vi "VI-File-Explorer.vi"() -> ()   [LabVIEW 2016, in "vi_lib.lvlib"]
uses:
  vi_lib.lvlib
  clLabview/clLabview.lvclass
  clFile/clFile.lvclass
panel:
  in  "new VI-Lib Password":string
  in  "Update LV-Lib Password":bool
  out "File is protected?":bool=TRUE
  out "LV-Lib password (Hex)":string
  out "Icon":picture
  out "busy (*)":bool
  out "Salt (Hex)":string
  out "MD5-Hash 2 (Hex)":string
  out "MD5-Hash 1 (Hex)":string
  out "saving done":bool
  in  "Save":bool
  in  "Open":bool
  in  "stop":bool
  out "flags":i32 step=1
  out "stage":u8(ring) items=["development", "alpha", "beta", "release"]
  out "build":u8 step=1
  out "bugfix":u8 step=1
  out "minor":u8 max=99 step=1
  out "major":u8=3 min=1 max=99 step=1
  out "version info":string
  out "version text":string
  in  "save to":path=path "D:/labview/file_in_(free).vi"
  in  "new File Password":string
  in  "open from":path
  out "MD5 password (Hex)":string
  # "File password [BDPW]"
  # "VI-File Explorer v.0.9"
  # "by Thomas Zeugner"
  # "Please report bugs and comments to: TomSoftware@gmx.de"
  # "Open"
  # "for LV-Version >= 8"
  # "for LV-Version >= 12"
  # "Save"
  # "File propertys [LVSR]"
  # "File version [vers]"
  # "(*) This is a \"brute force\" version to calc the password Salt, \n      so it might take up to 30sec."
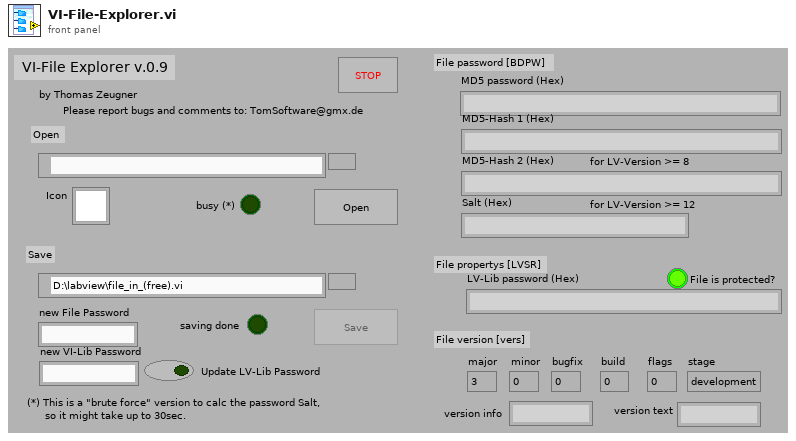
[diagram p1: front panel]
types:
  T1 = enum8{"Enabled", "Disabled", "Disabled and Grayed Out"}
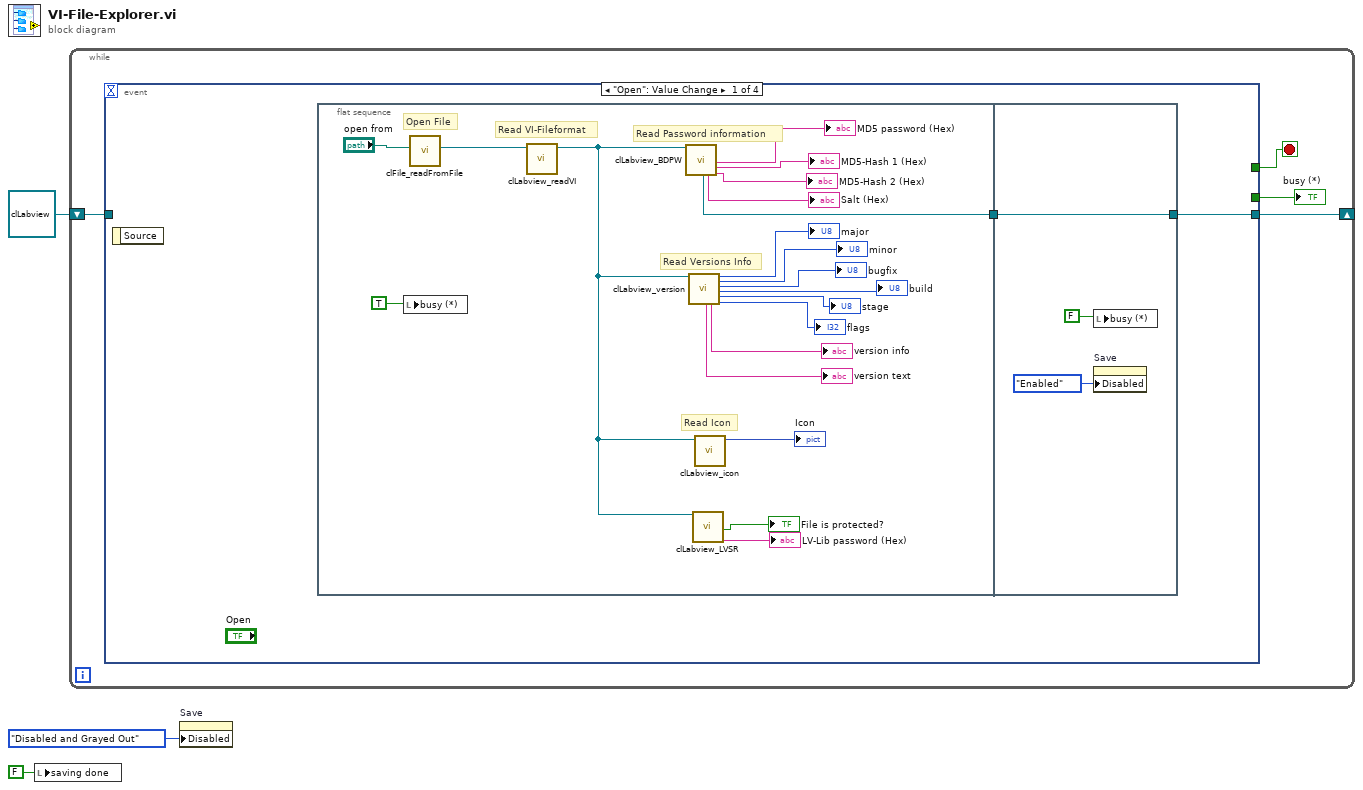
[diagram p0: block diagram]
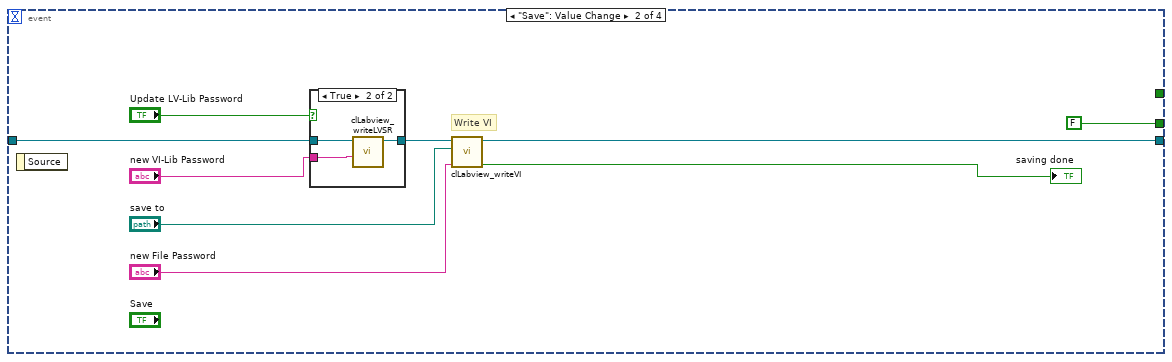
[diagram p2: hidden frame]
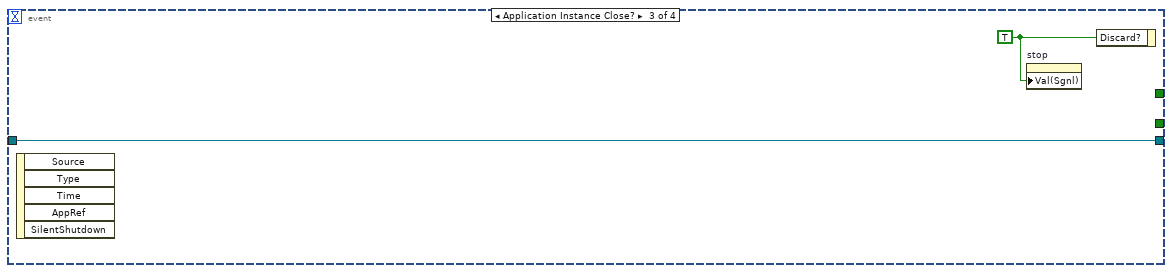
[diagram p4: hidden frame]
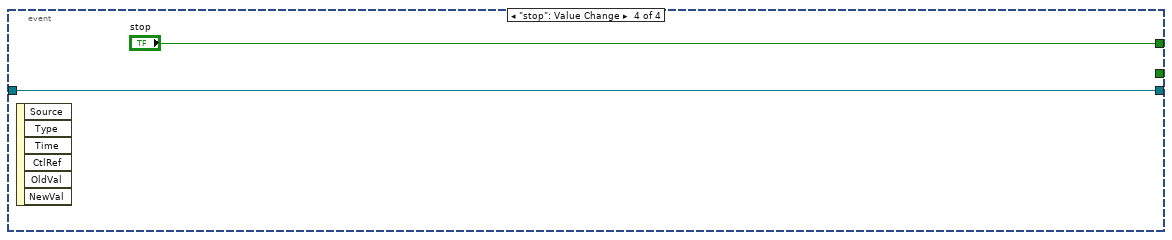
[diagram p5: hidden frame]
diagram:
  n1 = local write "saving done"(FALSE ("saving done")) -> ()
  n2 = while {
    shift-right: [w6] -> _
    shift-left: refnum<class "clLabview.lvclass"> refnum ("vi_lib.lvlib:clLabview.lvclass 2") -> [w7]
    stop <- w4 stop-if-true
    n3 = event shown="[0] \"Open\": Value Change" {
      selector: _ -> [_ _ _ _]
      dyn-events: _ -> [_ _ _ _]
      timeout: _ -> [_ _ _ _]
      tunnel: w7 -> [_ w35 w46 w48]
      tunnel: [w8 w34 w46 w48] -> w6
      tunnel: [_ FALSE ("busy") _ _] -> w5
      tunnel: [_ _ _ "stop"] -> w4
      event "Open": Value Change {
        n4 = event-data() -> ()  [unwired: 1 in, 1 out]
        n5 = flat-sequence {
          tunnel: [w15] -> w9
          tunnel: [w32] -> w8
          tunnel: w9 -> [w32]
          frame #0 {
            # "Read Icon"
            # "Read Versions Info"
            # "Read Password information"
            # "Read VI-Fileformat"
            # "Open File"
            n6 = local write "busy (*)"(TRUE ("busy")) -> ()
            n7 = call "clFile_readFromFile.vi"("file (use dialog)"="open from") -> ("clFileReader.lvclass"=w25:refnum<class "clFileReader.lvclass">)  [unwired: 1 in, 9 out]
            n8 = call "clLabview_readVI.vi"("vi_lib.lvlib:clFileReader.lvclass"=w25) -> ("vi_lib.lvlib:clLabview.lvclass 2"=w12:refnum<class "clLabview.lvclass">)  [unwired: 10 out]
            n9 = call "clLabview_BDPW.vi"("vi_lib.lvlib:clLabview.lvclass"=w12) -> ("vi_lib.lvlib:clLabview.lvclass [Out]"=w15:refnum<class "clLabview.lvclass">, "Salt (Hex)"=→"Salt (Hex)":string, "MD5 password (Hex)"=→"MD5 password (Hex)":string, "MD5-Hash 1  (Hex)"=→"MD5-Hash 1 (Hex)":string, "MD5-Hash 2  (Hex)"=→"MD5-Hash 2 (Hex)":string)  [unwired: 14 out]
            n10 = call "clLabview_version.vi"("vi_lib.lvlib:clLabview.lvclass"=w12) -> ("version_text"=→"version text":string, "version_info"=→"version info":string, "major"=→"major":u8, "minor"=→"minor":u8, "bugfix"=→"bugfix":u8, "build"=→"build":u8, "stage"=→"stage":u8, "flags"=→"flags":i32)  [unwired: 11 out]
            n11 = call "clLabview_LVSR.vi"("vi_lib.lvlib:clLabview.lvclass"=w12) -> ("File is protected?"=→"File is protected?":bool, "MD5 lib Password (Hex)"=→"LV-Lib password (Hex)":string)  [unwired: 17 out]
            n12 = call "clLabview_icon.vi"("vi_lib.lvlib:clLabview.lvclass"=w12) -> ("Icon"=→"Icon":picture)  [unwired: 10 out]
          }
          frame #1 {
            n13 = local write "busy (*)"(FALSE ("busy")) -> ()
            n14 = property on="Save" class="Bool"("Disabled"=T1."Enabled") -> ()  [unwired: 2 in, 2 out]
          }
        }
      }
      event "Save": Value Change {
        # "Write VI"
        n15 = event-data() -> ()  [unwired: 1 in, 1 out]
        n16 = case shown="True" "Update LV-Lib Password" {
          tunnel: w35 -> [w42 w45]
          tunnel: [w42 w44] -> w38
          tunnel: "new VI-Lib Password" -> [_ w43]
          frame False {
          }
          frame True {
            n17 = call "clLabview_writeLVSR.vi"("vi_lib.lvlib:clLabview.lvclass"=w45, "new lib Password"=w43) -> ("vi_lib.lvlib:clLabview.lvclass [Out]"=w44:refnum<class "clLabview.lvclass">)  [unwired: 8 out]
          }
        }
        n18 = call "clLabview_writeVI.vi"("vi_lib.lvlib:clLabview.lvclass"=w38, "filename (use dialog)"="save to", "new Password"="new File Password") -> ("vi_lib.lvlib:clLabview.lvclass [Out]"=w34:refnum<class "clLabview.lvclass">, "no Error"=→"saving done":bool)  [unwired: 6 out]
      }
      event Application Instance Close? {
        w47 = TRUE ("Discard?")
        n19 = event-data() -> ()  [unwired: 1 in, 5 out]
        n20 = property on="stop" class="Bool (strict)"("Val(Sgnl)"=w47) -> ()  [unwired: 2 in, 2 out]
        n21 = event-data("Discard?"=w47) -> ()  [unwired: 1 in, 1 out]
      }
      event "stop": Value Change {
        n22 = event-data() -> ()  [unwired: 1 in, 6 out]
      }
    }
    "busy (*)" <- w5
  }
  n23 = property on="Save" class="Bool"("Disabled"=T1."Disabled and Grayed Out") -> ()  [unwired: 2 in, 2 out]
